vi "Calendar (LabVIEW 2021).vi"(0 "Calendar Type":enum32{"Persian", "Gregorian", "Hijri"}(radio)) -> (1 "Persian Year":i32 format="%04d", 4 "Persian Month":i32 format="%02d", 5 "Persian Day":i32 format="%02d", 6 "Gregorian Year":i32 format="%04d", 7 "Gregorian Month":i32 format="%02d", 11 "Formatted Output":string, 12 "Gregorian Day":i32 format="%02d", 13 "Hour":i32 format="%02d", 14 "Minute":i32 format="%02d", 15 "Second":i32 format="%02d", 16 "Raw Output":string, 17 "Persian Month Name":string, 18 "Date String":string, 19 "Time String":string)   [LabVIEW 2021]
panel:
  out "Hijri Month Name":string
  out "Hijri Day":i32 format="%02d"
  out "Hijri Month":i32 format="%02d"
  out "Hijri Year":i32 format="%04d"
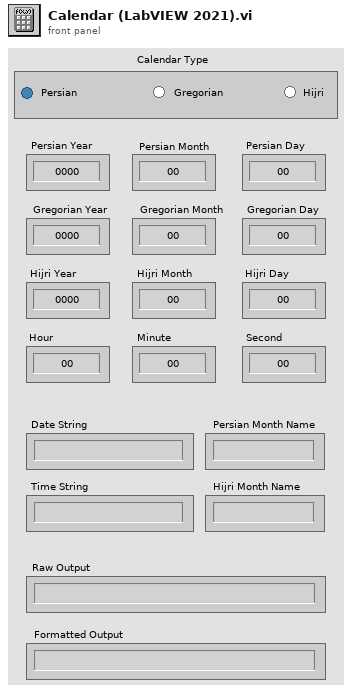
[diagram p1: front panel]
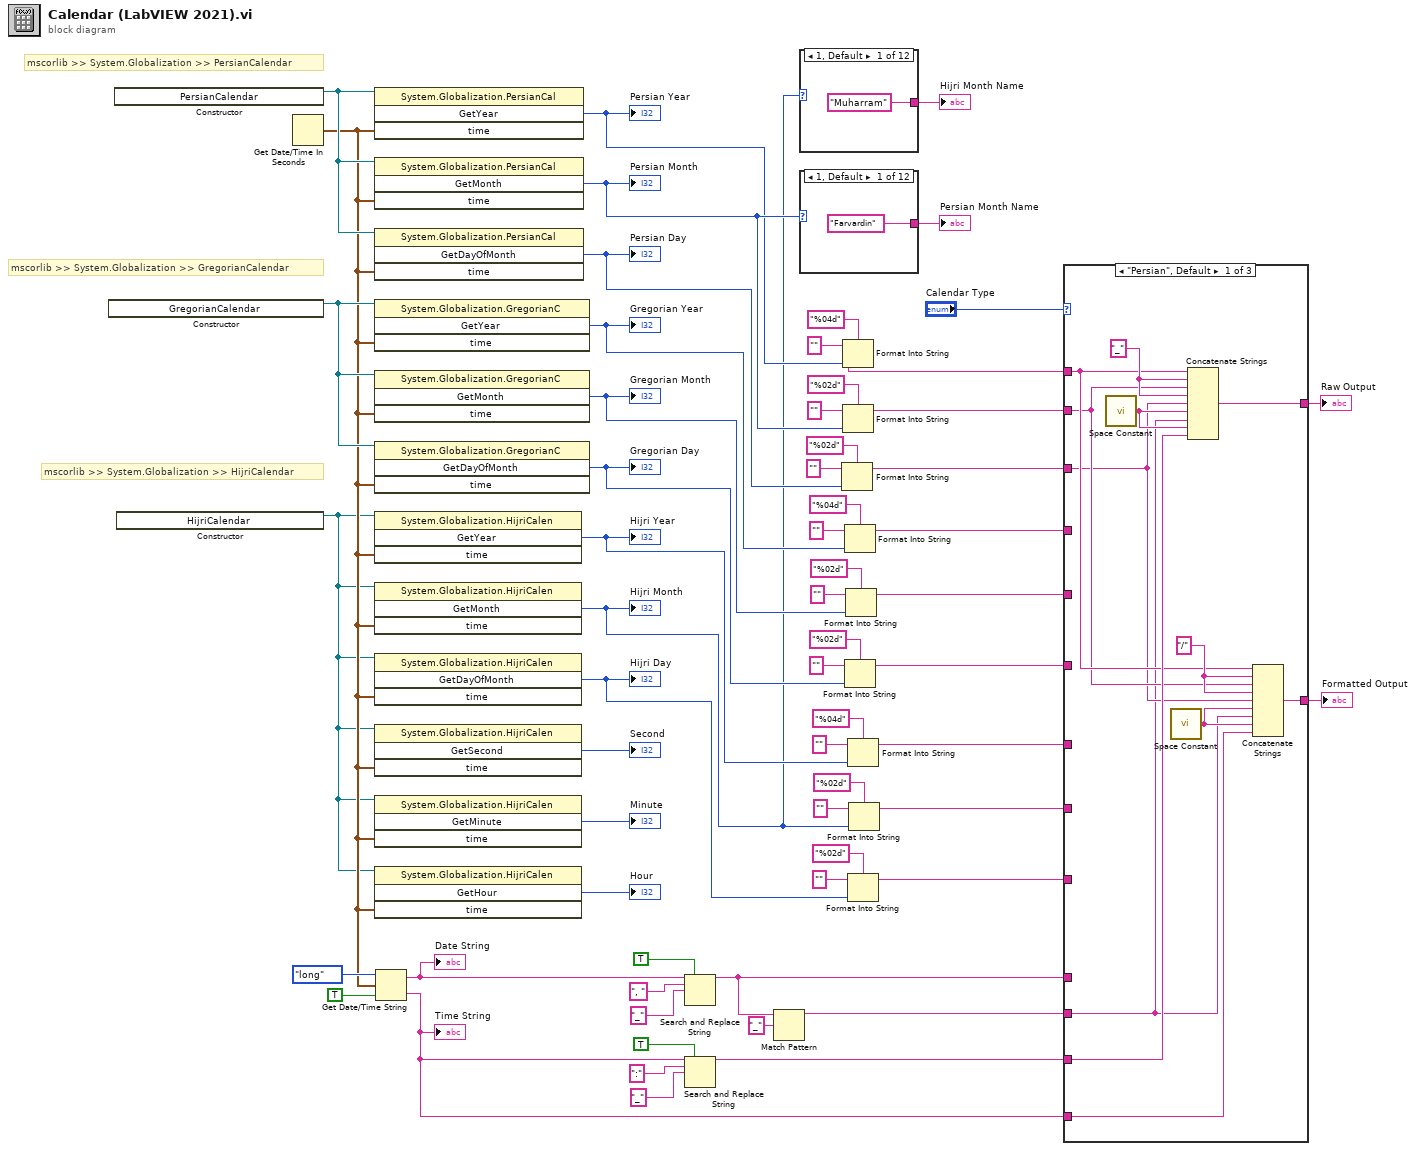
[diagram p0: block diagram]
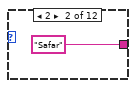
[diagram p2: hidden frame]
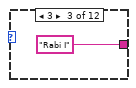
[diagram p3: hidden frame]
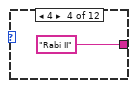
[diagram p4: hidden frame]
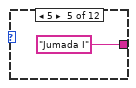
[diagram p5: hidden frame]
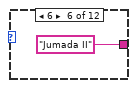
[diagram p6: hidden frame]
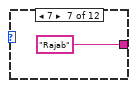
[diagram p7: hidden frame]
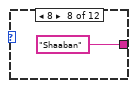
[diagram p8: hidden frame]
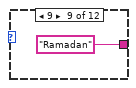
[diagram p9: hidden frame]
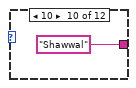
[diagram p10: hidden frame]
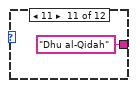
[diagram p11: hidden frame]
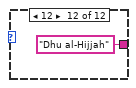
[diagram p12: hidden frame]
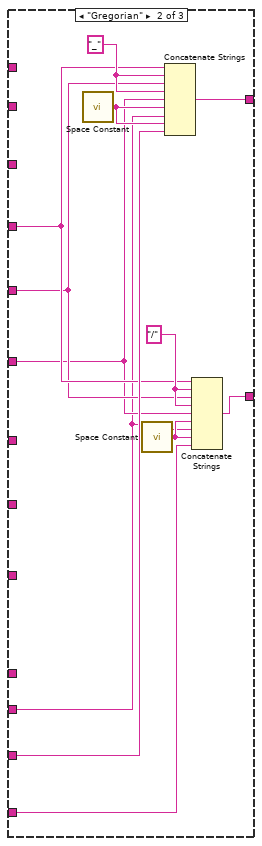
[diagram p13: hidden frame]
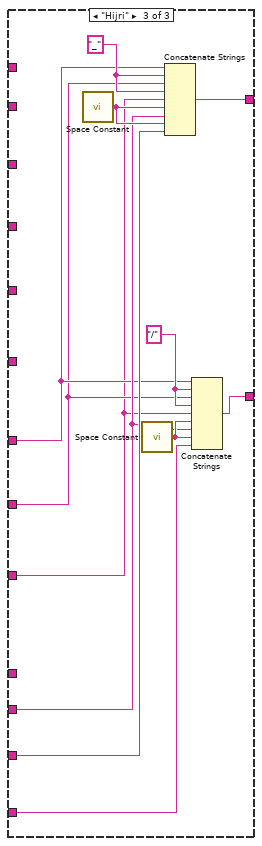
[diagram p14: hidden frame]
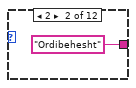
[diagram p15: hidden frame]
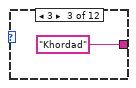
[diagram p16: hidden frame]
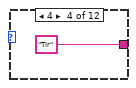
[diagram p17: hidden frame]
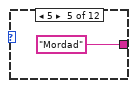
[diagram p18: hidden frame]
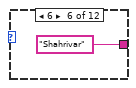
[diagram p19: hidden frame]
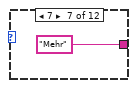
[diagram p20: hidden frame]
diagram:
  # "mscorlib >> System.Globalization >> HijriCalendar"
  # "mscorlib >> System.Globalization >> GregorianCalendar"
  # "mscorlib >> System.Globalization >> PersianCalendar"
  n1 = constructor class="System.Globalization.GregorianC"() -> (reference out=w61:refnum<k24>)  [unwired: 3 in, 2 out]
  n2 = constructor class="System.Globalization.PersianCal"() -> (reference out=w62:refnum<k24>)  [unwired: 3 in, 2 out]
  n3 = constructor class="System.Globalization.HijriCalen"() -> (reference out=w14:refnum<k24>)  [unwired: 3 in, 2 out]
  n4 = Get Date/Time In Seconds() -> (seconds since 1Jan1904=w17:timestamp)
  n5 = invoke class="System.Globalization.PersianCal" method="GetYear"(reference=w62, "time"=w17) -> ("GetYear"=w38:i32)  [unwired: 2 in, 3 out]
  "Persian Year" <- w38
  n6 = invoke class="System.Globalization.PersianCal" method="GetMonth"(reference=w62, "time"=w17) -> ("GetMonth"=w41:i32)  [unwired: 2 in, 3 out]
  "Persian Month" <- w41
  n7 = invoke class="System.Globalization.PersianCal" method="GetDayOfMonth"(reference=w62, "time"=w17) -> ("GetDayOfMonth"=w32:i32)  [unwired: 2 in, 3 out]
  "Persian Day" <- w32
  n8 = invoke class="System.Globalization.GregorianC" method="GetYear"(reference=w61, "time"=w17) -> ("GetYear"=w22:i32)  [unwired: 2 in, 3 out]
  "Gregorian Year" <- w22
  n9 = invoke class="System.Globalization.GregorianC" method="GetMonth"(reference=w61, "time"=w17) -> ("GetMonth"=w21:i32)  [unwired: 2 in, 3 out]
  "Gregorian Month" <- w21
  n10 = invoke class="System.Globalization.GregorianC" method="GetDayOfMonth"(reference=w61, "time"=w17) -> ("GetDayOfMonth"=w20:i32)  [unwired: 2 in, 3 out]
  "Gregorian Day" <- w20
  n11 = invoke class="System.Globalization.HijriCalen" method="GetYear"(reference=w14, "time"=w17) -> ("GetYear"=w7:i32)  [unwired: 2 in, 3 out]
  "Hijri Year" <- w7
  n12 = invoke class="System.Globalization.HijriCalen" method="GetMonth"(reference=w14, "time"=w17) -> ("GetMonth"=w1:i32)  [unwired: 2 in, 3 out]
  "Hijri Month" <- w1
  n13 = invoke class="System.Globalization.HijriCalen" method="GetDayOfMonth"(reference=w14, "time"=w17) -> ("GetDayOfMonth"=w6:i32)  [unwired: 2 in, 3 out]
  "Hijri Day" <- w6
  n14 = invoke class="System.Globalization.HijriCalen" method="GetSecond"(reference=w14, "time"=w17) -> ("GetSecond"=→"Second":i32)  [unwired: 2 in, 3 out]
  n15 = invoke class="System.Globalization.HijriCalen" method="GetMinute"(reference=w14, "time"=w17) -> ("GetMinute"=→"Minute":i32)  [unwired: 2 in, 3 out]
  n16 = invoke class="System.Globalization.HijriCalen" method="GetHour"(reference=w14, "time"=w17) -> ("GetHour"=→"Hour":i32)  [unwired: 2 in, 3 out]
  n17 = Get Date/Time String(date format (0)=enum16{"short", "long", "abbreviated"}."long", seconds (now)=w17, want seconds? (F)=TRUE) -> (date string=w19:string, time string=w15:string)
  "Date String" <- w19
  "Time String" <- w15
  n18 = Search and Replace String(replace all?=TRUE ("replace all? (F)"), input string=w19, search string=", " ("substring (\"\")"), replace string="_" ("replace string (\"\")")) -> (result string=w16:string)  [unwired: 4 in, 3 out]
  n19 = Search and Replace String(replace all?=TRUE ("replace all? (F)"), input string=w15, search string=":" ("substring (\"\")"), replace string="_" ("replace string (\"\")")) -> (result string=w47:string)  [unwired: 4 in, 3 out]
  n20 = Match Pattern(string=w16, regular expression="_") -> (before substring=w45:string)  [unwired: 1 in, 3 out]
  n21 = case shown="1, Default" w1 {
    tunnel: ["Muharram" "Safar" "Rabi I" "Rabi II" "Jumada I" "Jumada II" "Rajab" "Shaaban" "Ramadan" "Shawwal" "Dhu al-Qidah" "Dhu al-Hijjah"] -> w2
    frame 1, Default {
    }
    frame 2 {
    }
    frame 3 {
    }
    frame 4 {
    }
    frame 5 {
    }
    frame 6 {
    }
    frame 7 {
    }
    frame 8 {
    }
    frame 9 {
    }
    frame 10 {
    }
    frame 11 {
    }
    frame 12 {
    }
  }
  "Hijri Month Name" <- w2
  n22 = case shown="1, Default" w41 {
    tunnel: ["Farvardin" "Ordibehesht" "Khordad" "Tir" "Mordad" "Shahrivar" "Mehr" "Aban" "Azar" "Dey" "Bahman" "Esfand"] -> w58
    frame 1, Default {
    }
    frame 2 {
    }
    frame 3 {
    }
    frame 4 {
    }
    frame 5 {
    }
    frame 6 {
    }
    frame 7 {
    }
    frame 8 {
    }
    frame 9 {
    }
    frame 10 {
    }
    frame 11 {
    }
    frame 12 {
    }
  }
  "Persian Month Name" <- w58
  n23 = Format Into String(format string="%02d", initial string="", w32) -> (resulting string=w33:string)  [unwired: 1 in, 1 out]
  n24 = Format Into String(format string="%04d", initial string="", w38) -> (resulting string=w37:string)  [unwired: 1 in, 1 out]
  n25 = Format Into String(format string="%02d", initial string="", w41) -> (resulting string=w43:string)  [unwired: 1 in, 1 out]
  n26 = Format Into String(format string="%04d", initial string="", w22) -> (resulting string=w25:string)  [unwired: 1 in, 1 out]
  n27 = Format Into String(format string="%02d", initial string="", w20) -> (resulting string=w23:string)  [unwired: 1 in, 1 out]
  n28 = Format Into String(format string="%02d", initial string="", w21) -> (resulting string=w24:string)  [unwired: 1 in, 1 out]
  n29 = Format Into String(format string="%04d", initial string="", w7) -> (resulting string=w5:string)  [unwired: 1 in, 1 out]
  n30 = Format Into String(format string="%02d", initial string="", w6) -> (resulting string=w3:string)  [unwired: 1 in, 1 out]
  n31 = Format Into String(format string="%02d", initial string="", w1) -> (resulting string=w4:string)  [unwired: 1 in, 1 out]
  n32 = case shown="\"Persian\", Default" "Calendar Type" {
    tunnel: w16 -> [_ _ _]
    tunnel: w47 -> [w98 w110 w122]
    tunnel: w37 -> [w92 _ _]
    tunnel: w43 -> [w91 _ _]
    tunnel: w33 -> [w90 _ _]
    tunnel: w25 -> [_ w104 _]
    tunnel: w24 -> [_ w103 _]
    tunnel: w23 -> [_ w102 _]
    tunnel: w45 -> [w89 w99 w114]
    tunnel: [w97 w109 w121] -> w44
    tunnel: w15 -> [w88 w101 w116]
    tunnel: [w87 w100 w115] -> w18
    tunnel: w5 -> [_ _ w113]
    tunnel: w4 -> [_ _ w112]
    tunnel: w3 -> [_ _ w111]
    frame "Persian", Default {
      w93 = "/"
      w96 = "_"
      n33 = call <vilib>:"Space Constant.vi"() -> ("String"=w95:string)
      n34 = call <vilib>:"Space Constant.vi"() -> ("String"=w94:string)
      n35 = Concatenate Strings(w92, w96, w91, w96, w90, w95, w89, w95, w98) -> (w97:string)
      n36 = Concatenate Strings(w92, w93, w91, w93, w90, w94, w89, w94, w88) -> (w87:string)
    }
    frame "Gregorian" {
      w105 = "/"
      w108 = "_"
      n37 = call <vilib>:"Space Constant.vi"() -> ("String"=w107:string)
      n38 = call <vilib>:"Space Constant.vi"() -> ("String"=w106:string)
      n39 = Concatenate Strings(w104, w108, w103, w108, w102, w107, w99, w107, w110) -> (w109:string)
      n40 = Concatenate Strings(w104, w105, w103, w105, w102, w106, w99, w106, w101) -> (w100:string)
    }
    frame "Hijri" {
      w117 = "/"
      w120 = "_"
      n41 = call <vilib>:"Space Constant.vi"() -> ("String"=w119:string)
      n42 = call <vilib>:"Space Constant.vi"() -> ("String"=w118:string)
      n43 = Concatenate Strings(w113, w120, w112, w120, w111, w119, w114, w119, w122) -> (w121:string)
      n44 = Concatenate Strings(w113, w117, w112, w117, w111, w118, w114, w118, w116) -> (w115:string)
    }
  }
  "Raw Output" <- w44
  "Formatted Output" <- w18
